vi "SP_OEE_2_test.vi"() -> ()   [LabVIEW 2017] (continued)
                        w9152 = string[] [""]
                        n1667 = Insert Into Array(array=w9162, index (col)=1 ("disabled index (col)"), new element #1=w9152, new element #2=w9152, new element #3=w9152, new element #4=w9152, new element #5=w9152, new element #6=w9152, new element #7=w9152, new element #8=w9152, new element #9=w9153, new element #10=w9154, new element #11=w9155, new element #12=w9156) -> (w9158:string[][])  [unwired: 1 in]
                        n1668 = call "flot graph for month n year.vi"("BD Date"=w9159, "error in (no error)"=w9161, "Count total"=w9155) -> ("error out"=w9160:errorcluster, "Run-Time Status"=w9157:cluster{"Array 2":timestamp[], dbl[]})  [unwired: 7 in]
                        n1669 = local write "Run-Time Status"(w9157) -> ()
                        n1670 = local write "Table"(w9158) -> ()
                      }
                    }
                  }
                  frame "all" {
                  }
                }
              }
            }
          }
          frame "STATION 1" {
            (unwired) "ALL" ("Select Stakeholder")
            n1671 = case shown="\"ALL\"" "ALL" {
              tunnel: w9178 -> [_ w9192 w10652 w12131 w13625 w15132 w16654]
              tunnel: w9177 -> [_ w9191 w10651 w12130 w13624 w15131 w16653]
              tunnel: w9176 -> [_ w9190 w10650 w12129 w13623 w15130 w16652]
              tunnel: w9175 -> [_ w9189 w10649 w12128 w13622 w15129 w16651]
              tunnel: w9174 -> [_ w9188 w10648 w12127 w13621 w15128 w16650]
              tunnel: [_ w9185 _ w12125 _ _ _] -> w9173
              tunnel: [_ w9186 _ w12124 _ _ _] -> w9172
              tunnel: w9170 -> [_ w9184 _ _ _ _ _]
              tunnel: w9169 -> [_ w9183 _ _ _ _ _]
              tunnel: w9168 -> [_ w9182 _ _ _ _ _]
              tunnel: w9167 -> [_ w9181 _ _ _ _ _]
              tunnel: w9166 -> [_ w9180 _ _ _ _ _]
              tunnel: w9165 -> [_ w9179 _ _ _ _ _]
              frame "False", Default {
              }
              frame "ALL" {
                n1672 = local read "Shift"() -> (w9187:string)
                n1673 = case shown="\"ALL\", Default" w9187 {
                  selector: w9187 -> [_ w9568 w9935 w10302 _]
                  tunnel: w9192 -> [w9218 w9577 w9944 w10311 _]
                  tunnel: w9191 -> [w9217 w9576 w9943 w10310 _]
                  tunnel: w9190 -> [w9216 w9575 w9942 w10309 _]
                  tunnel: w9189 -> [w9215 w9574 w9941 w10308 _]
                  tunnel: w9188 -> [w9214 w9573 w9940 w10307 _]
                  tunnel: [w9199 w9553 w9920 w10287 _] -> w9186
                  tunnel: [w9209 w9552 w9919 w10286 _] -> w9185
                  tunnel: w9184 -> [w9207 w9558 w9924 w10293 _]
                  tunnel: w9183 -> [w9206 w9557 w9923 w10292 _]
                  tunnel: w9182 -> [w9205 w9560 w9928 w10295 _]
                  tunnel: w9181 -> [w9204 w9559 w9927 w10294 _]
                  tunnel: w9180 -> [w9202 w9556 w9925 w10290 _]
                  tunnel: w9179 -> [w9201 w9555 w9922 w10289 _]
                  frame "ALL", Default {
                    n1674 = flat-sequence {
                      tunnel: w9218 -> [w9330]
                      tunnel: w9217 -> [w9328]
                      tunnel: [w9314] -> w9308
                      tunnel: [w9329] -> w9307
                      tunnel: w9216 -> [_]
                      tunnel: [w9333] -> w9306
                      tunnel: [w9313] -> w9305
                      tunnel: [w9312] -> w9304
                      tunnel: [w9311] -> w9303
                      tunnel: w9215 -> [w9313]
                      tunnel: w9214 -> [w9312]
                      tunnel: ["Where BREAKDOWN_DATE between '%s'and '%s' and BREAKDOWN_STK_HOLD_ID ='%d' and STATION_ID_CID_TRIGGER =%d "] -> w9302
                      tunnel: [w9311] -> w9301
                      tunnel: w9308 -> [w9394]
                      tunnel: w9307 -> [w9396]
                      tunnel: w9306 -> [w9391]
                      tunnel: w9305 -> [w9390]
                      tunnel: w9304 -> [w9389]
                      tunnel: [w9393] -> w9300
                      tunnel: [w9395] -> w9299
                      tunnel: [w9391] -> w9298
                      tunnel: [w9381] -> w9297
                      tunnel: [w9387] -> w9296
                      tunnel: [w9390] -> w9295
                      tunnel: [w9389] -> w9294
                      tunnel: w9303 -> [w9386]
                      tunnel: [w9386] -> w9293
                      tunnel: w9302 -> [w9383]
                      tunnel: [w9383] -> w9292
                      tunnel: [w9382] -> w9291
                      tunnel: w9301 -> [w9382]
                      tunnel: [w9380] -> w9213
                      tunnel: w9300 -> [w9412]
                      tunnel: w9299 -> [w9410]
                      tunnel: w9298 -> [w9415]
                      tunnel: w9297 -> [w9414]
                      tunnel: w9296 -> [w9413]
                      tunnel: w9295 -> [w9407]
                      tunnel: w9294 -> [w9406]
                      tunnel: [w9415] -> w9290
                      tunnel: [w9414] -> w9289
                      tunnel: [w9413] -> w9288
                      tunnel: [w9411] -> w9287
                      tunnel: [w9404] -> w9286
                      tunnel: [w9403] -> w9285
                      tunnel: [w9408] -> w9284
                      tunnel: [w9407] -> w9283
                      tunnel: [w9406] -> w9282
                      tunnel: w9293 -> [w9402]
                      tunnel: [w9402] -> w9281
                      tunnel: w9292 -> [w9399]
                      tunnel: [w9399] -> w9280
                      tunnel: [w9398] -> w9279
                      tunnel: w9291 -> [w9398]
                      tunnel: w9213 -> [w9397]
                      tunnel: [w9397] -> w9212
                      tunnel: w9290 -> [w9436]
                      tunnel: w9289 -> [w9435]
                      tunnel: w9288 -> [w9434]
                      tunnel: w9287 -> [w9430]
                      tunnel: w9286 -> [w9433]
                      tunnel: w9285 -> [w9432]
                      tunnel: w9284 -> [w9428]
                      tunnel: w9283 -> [w9426]
                      tunnel: w9282 -> [w9425]
                      tunnel: [w9436] -> w9278
                      tunnel: [w9435] -> w9277
                      tunnel: [w9434] -> w9276
                      tunnel: [w9433] -> w9275
                      tunnel: [w9432] -> w9274
                      tunnel: [w9429] -> w9273
                      tunnel: [w9423] -> w9272
                      tunnel: [w9422] -> w9271
                      tunnel: [w9427] -> w9270
                      tunnel: [w9426] -> w9269
                      tunnel: [w9425] -> w9268
                      tunnel: w9281 -> [w9421]
                      tunnel: [w9421] -> w9267
                      tunnel: w9280 -> [w9418]
                      tunnel: [w9418] -> w9266
                      tunnel: [w9417] -> w9265
                      tunnel: w9279 -> [w9417]
                      tunnel: w9212 -> [w9416]
                      tunnel: [w9416] -> w9211
                      tunnel: w9278 -> [w9459]
                      tunnel: w9277 -> [w9458]
                      tunnel: w9276 -> [w9457]
                      tunnel: w9275 -> [w9456]
                      tunnel: w9274 -> [w9455]
                      tunnel: w9273 -> [w9451]
                      tunnel: w9272 -> [w9454]
                      tunnel: w9271 -> [w9453]
                      tunnel: w9270 -> [w9450]
                      tunnel: w9269 -> [w9447]
                      tunnel: w9268 -> [w9446]
                      tunnel: [w9459] -> w9264
                      tunnel: [w9458] -> w9263
                      tunnel: [w9457] -> w9262
                      tunnel: [w9456] -> w9261
                      tunnel: [w9455] -> w9260
                      tunnel: [w9454] -> w9259
                      tunnel: [w9453] -> w9258
                      tunnel: [w9449] -> w9257
                      tunnel: [w9448] -> w9256
                      tunnel: [w9444] -> w9255
                      tunnel: [w9443] -> w9254
                      tunnel: [w9447] -> w9253
                      tunnel: [w9446] -> w9252
                      tunnel: w9267 -> [w9442]
                      tunnel: [w9442] -> w9251
                      tunnel: w9266 -> [w9439]
                      tunnel: [w9439] -> w9250
                      tunnel: [w9438] -> w9249
                      tunnel: w9265 -> [w9438]
                      tunnel: w9211 -> [w9437]
                      tunnel: [w9437] -> w9210
                      tunnel: w9264 -> [w9484]
                      tunnel: w9263 -> [w9483]
                      tunnel: w9262 -> [w9482]
                      tunnel: w9261 -> [w9481]
                      tunnel: w9260 -> [w9480]
                      tunnel: w9259 -> [w9479]
                      tunnel: w9258 -> [w9478]
                      tunnel: w9257 -> [w9472]
                      tunnel: w9256 -> [w9474]
                      tunnel: w9255 -> [w9477]
                      tunnel: w9254 -> [w9476]
                      tunnel: w9253 -> [w9469]
                      tunnel: w9252 -> [w9470]
                      tunnel: [w9484] -> w9248
                      tunnel: [w9483] -> w9247
                      tunnel: [w9482] -> w9246
                      tunnel: [w9481] -> w9245
                      tunnel: [w9480] -> w9244
                      tunnel: [w9479] -> w9243
                      tunnel: [w9478] -> w9242
                      tunnel: [w9477] -> w9241
                      tunnel: [w9476] -> w9240
                      tunnel: [w9473] -> w9239
                      tunnel: [w9471] -> w9238
                      tunnel: [w9467] -> w9237
                      tunnel: [w9465] -> w9236
                      tunnel: w9251 -> [w9466]
                      tunnel: w9250 -> [w9462]
                      tunnel: [w9461] -> w9235
                      tunnel: w9249 -> [w9461]
                      tunnel: w9210 -> [w9460]
                      tunnel: w9248 -> [w9511]
                      tunnel: w9247 -> [w9504]
                      tunnel: w9246 -> [w9495]
                      tunnel: w9245 -> [w9503]
                      tunnel: w9244 -> [w9493]
                      tunnel: w9243 -> [w9502]
                      tunnel: w9242 -> [w9491]
                      tunnel: w9241 -> [w9501]
                      tunnel: w9240 -> [w9489]
                      tunnel: w9239 -> [w9525]
                      tunnel: w9238 -> [w9524]
                      tunnel: w9237 -> [w9500]
                      tunnel: w9236 -> [w9487]
                      tunnel: [w9525] -> w9234
                      tunnel: [w9524] -> w9233
                      tunnel: [w9518] -> w9232
                      tunnel: [w9511] -> w9231
                      tunnel: [w9510] -> w9230
                      tunnel: [w9509] -> w9229
                      tunnel: [w9508] -> w9228
                      tunnel: [w9507] -> w9227
                      tunnel: [w9506] -> w9226
                      tunnel: [w9505] -> w9225
                      tunnel: [w9504] -> w9224
                      tunnel: [w9503] -> w9223
                      tunnel: [w9502] -> w9222
                      tunnel: [w9501] -> w9221
                      tunnel: [w9500] -> w9220
                      tunnel: [w9485] -> w9219
                      tunnel: w9235 -> [w9485]
                      tunnel: [w9545] -> w9200
                      tunnel: [w9531] -> w9209
                      tunnel: w9234 -> [w9532]
                      tunnel: w9233 -> [w9545]
                      tunnel: w9232 -> [w9530]
                      tunnel: w9231 -> [w9543]
                      tunnel: w9230 -> [w9541]
                      tunnel: w9229 -> [w9539]
                      tunnel: w9228 -> [w9537]
                      tunnel: w9227 -> [w9535]
                      tunnel: w9226 -> [w9533]
                      tunnel: w9225 -> [w9526]
                      tunnel: w9224 -> [w9542]
                      tunnel: w9223 -> [w9540]
                      tunnel: w9222 -> [w9538]
                      tunnel: w9221 -> [w9536]
                      tunnel: w9220 -> [w9534]
                      tunnel: w9219 -> [w9529]
                      tunnel: [w9526] -> w9203
                      frame #0 {
                        w9321 = "%Y-%m-%d" ("time format string (%c)")
                        n1675 = property on="Table" class="Tbl (strict)"("Visible"=TRUE) -> ()  [unwired: 2 in, 2 out]
                        n1676 = Format Date/Time String(time format string (%c)=w9321, seconds (now)=w9313) -> (date/time string=w9322:string)  [unwired: 1 in]
                        n1677 = Format Date/Time String(time format string (%c)=w9321, seconds (now)=w9312) -> (date/time string=w9320:string)  [unwired: 1 in]
                        n1678 = Format Into String(format string="Where BREAKDOWN_DATE between '%s' and '%s' ", w9322, w9320) -> (resulting string=w9319:string)  [unwired: 2 in, 1 out]
                        n1679 = call <vilib>:"DB Tools Select Data.vi"("condition"=w9319, "error in (no error)"=w9328, "columns"=string[] ["BREAKDOWN_DATE"], "table"="STATION_1_LOG_HISTORY", "connection reference"=w9330) -> ("error out"=w9315:errorcluster, "data"=w9318:variant[][], "connection reference out"=w9329:T2)  [unwired: 1 in]
                        n1680 = property on="Table 2" class="Tbl (strict)"("Visible"=FALSE) -> ()  [unwired: 2 in, 2 out]
                        n1681 = xnode "Database Variant To Data"("database variant"=w9318, "error in (no error)"=w9315, "type"=string[][] [] ("Elements Found")) -> ("data"=w9316:string[][], "error out"=w9314:errorcluster)
                        n1682 = Index Array(array=w9316, index (col)=0 ("disabled index (col)")) -> (element=w9324:string[])  [unwired: 1 in]
                        n1683 = call "Search_1d_array_element.vi"("Count in"=string[] [] ("Elements Found"), "BD Date"=w9324, "Elements Found in"=string[] [] ("Elements Found")) -> ("Elements Found out"=w9311:string[])  [unwired: 4 in, 2 out]
                        n1684 = Build Array(w9311) -> (w9334:string[][])
                        n1685 = Transpose 2D Array(2D array=w9334) -> (transposed array=w9333:string[][])
                      }
                      frame #1 {
                        w9380 = 1 ("STATION_ID_CID_TRIGGER")
                        n1686 = call "Stack_holderwise_total_bd_count_&_duration_ST1.vi"("Refnum in"=w9396, "BREAKDOWN_STK_HOLD_ID"=1, "condition"=w9383, "Form Date"=w9390, "To Date"=w9389, "error in (no error)"=w9394, "STATION_ID_CID_TRIGGER"=w9380) -> ("Refnum out"=w9395:T2, "Count out"=w9388:string[], "appended array"=w9385:dbl[], "error out"=w9393:errorcluster)  [unwired: 5 in]
                        n1687 = call "NUMERIC TO STRING.vi"("appended array"=w9385) -> ("Array"=w9384:string[])  [unwired: 4 in]
                        n1688 = call "Insert_empty_element_with_zero.vi"("searched date"=w9388, "fixed date"=w9386) -> ("O/P"=w9381:string[])  [unwired: 9 in]
                        n1689 = call "Insert_empty_element_with_zero.vi"("searched date"=w9384, "fixed date"=w9386) -> ("O/P"=w9387:string[])  [unwired: 9 in]
                      }
                      frame #2 {
                        n1690 = call "Stack_holderwise_total_bd_count_&_duration_ST1.vi"("Refnum in"=w9410, "BREAKDOWN_STK_HOLD_ID"=2, "condition"=w9399, "Form Date"=w9407, "To Date"=w9406, "error in (no error)"=w9412, "STATION_ID_CID_TRIGGER"=w9397) -> ("Refnum out"=w9408:T2, "Count out"=w9405:string[], "appended array"=w9401:dbl[], "error out"=w9411:errorcluster)  [unwired: 5 in]
                        n1691 = call "Insert_empty_element_with_zero.vi"("searched date"=w9405, "fixed date"=w9402) -> ("O/P"=w9404:string[])  [unwired: 9 in]
                        n1692 = call "NUMERIC TO STRING.vi"("appended array"=w9401) -> ("Array"=w9400:string[])  [unwired: 4 in]
                        n1693 = call "Insert_empty_element_with_zero.vi"("searched date"=w9400, "fixed date"=w9402) -> ("O/P"=w9403:string[])  [unwired: 9 in]
                      }
                      frame #3 {
                        n1694 = call "Stack_holderwise_total_bd_count_&_duration_ST1.vi"("Refnum in"=w9428, "BREAKDOWN_STK_HOLD_ID"=3, "condition"=w9418, "Form Date"=w9426, "To Date"=w9425, "error in (no error)"=w9430, "STATION_ID_CID_TRIGGER"=w9416) -> ("Refnum out"=w9427:T2, "Count out"=w9424:string[], "appended array"=w9420:dbl[], "error out"=w9429:errorcluster)  [unwired: 5 in]
                        n1695 = call "Insert_empty_element_with_zero.vi"("searched date"=w9424, "fixed date"=w9421) -> ("O/P"=w9423:string[])  [unwired: 9 in]
                        n1696 = call "NUMERIC TO STRING.vi"("appended array"=w9420) -> ("Array"=w9419:string[])  [unwired: 4 in]
                        n1697 = call "Insert_empty_element_with_zero.vi"("searched date"=w9419, "fixed date"=w9421) -> ("O/P"=w9422:string[])  [unwired: 9 in]
                      }
                      frame #4 {
                        n1698 = call "Stack_holderwise_total_bd_count_&_duration_ST1.vi"("Refnum in"=w9450, "BREAKDOWN_STK_HOLD_ID"=4, "condition"=w9439, "Form Date"=w9447, "To Date"=w9446, "error in (no error)"=w9451, "STATION_ID_CID_TRIGGER"=w9437) -> ("Refnum out"=w9449:T2, "Count out"=w9445:string[], "appended array"=w9441:dbl[], "error out"=w9448:errorcluster)  [unwired: 5 in]
                        n1699 = call "Insert_empty_element_with_zero.vi"("searched date"=w9445, "fixed date"=w9442) -> ("O/P"=w9444:string[])  [unwired: 9 in]
                        n1700 = call "NUMERIC TO STRING.vi"("appended array"=w9441) -> ("Array"=w9440:string[])  [unwired: 4 in]
                        n1701 = call "Insert_empty_element_with_zero.vi"("searched date"=w9440, "fixed date"=w9442) -> ("O/P"=w9443:string[])  [unwired: 9 in]
                      }
                      frame #5 {
                        n1702 = call "Stack_holderwise_total_bd_count_&_duration_ST1.vi"("Refnum in"=w9472, "BREAKDOWN_STK_HOLD_ID"=5, "condition"=w9462, "Form Date"=w9469, "To Date"=w9470, "error in (no error)"=w9474, "STATION_ID_CID_TRIGGER"=w9460) -> ("Refnum out"=w9471:T2, "Count out"=w9468:string[], "appended array"=w9464:dbl[], "error out"=w9473:errorcluster)  [unwired: 5 in]
                        n1703 = call "NUMERIC TO STRING.vi"("appended array"=w9464) -> ("Array"=w9463:string[])  [unwired: 4 in]
                        n1704 = call "Insert_empty_element_with_zero.vi"("searched date"=w9468, "fixed date"=w9466) -> ("O/P"=w9467:string[])  [unwired: 9 in]
                        n1705 = call "Insert_empty_element_with_zero.vi"("searched date"=w9463, "fixed date"=w9466) -> ("O/P"=w9465:string[])  [unwired: 9 in]
                      }
                      frame #6 {
                        n1706 = call "String to numeric.vi"("Array"=w9495) -> ("Array 2"=w9494:dbl[])  [unwired: 4 in]
                        n1707 = call "String to numeric.vi"("Array"=w9493) -> ("Array 2"=w9492:dbl[])  [unwired: 4 in]
                        n1708 = call "String to numeric.vi"("Array"=w9491) -> ("Array 2"=w9490:dbl[])  [unwired: 4 in]
                        n1709 = call "String to numeric.vi"("Array"=w9489) -> ("Array 2"=w9488:dbl[])  [unwired: 4 in]
                        n1710 = call "String to numeric.vi"("Array"=w9487) -> ("Array 2"=w9486:dbl[])  [unwired: 4 in]
                        n1711 = Decimal String To Number(string=w9500) -> (number=w9519:i32[])  [unwired: 2 in, 1 out]
                        n1712 = Decimal String To Number(string=w9501) -> (number=w9520:i32[])  [unwired: 2 in, 1 out]
                        n1713 = Decimal String To Number(string=w9502) -> (number=w9521:i32[])  [unwired: 2 in, 1 out]
                        n1714 = Decimal String To Number(string=w9503) -> (number=w9522:i32[])  [unwired: 2 in, 1 out]
                        n1715 = Decimal String To Number(string=w9504) -> (number=w9517:i32[])  [unwired: 2 in, 1 out]
                        n1716 = Compound Arithmetic op=ADD(w9494, w9492, w9490, w9488, w9486) -> (w9497:dbl[])
                        n1717 = Build Array(w9495) -> (w9516:string[][])
                        n1718 = Build Array(w9493) -> (w9515:string[][])
                        n1719 = Build Array(w9491) -> (w9514:string[][])
                        n1720 = Build Array(w9489) -> (w9513:string[][])
                        n1721 = Build Array(w9487) -> (w9512:string[][])
                        n1722 = Number To Fractional String(number=w9497, precision (6)=i16 2) -> (F-format string=w9496:string[])  [unwired: 2 in]
                        n1723 = Compound Arithmetic op=ADD(w9519, w9520, w9521, w9522, w9517) -> (w9523:i32[])
                        n1724 = Transpose 2D Array(2D array=w9516) -> (transposed array=w9510:string[][])
                        n1725 = Transpose 2D Array(2D array=w9515) -> (transposed array=w9509:string[][])
                        n1726 = Transpose 2D Array(2D array=w9514) -> (transposed array=w9508:string[][])
                        n1727 = Transpose 2D Array(2D array=w9513) -> (transposed array=w9507:string[][])
                        n1728 = Transpose 2D Array(2D array=w9512) -> (transposed array=w9506:string[][])
                        n1729 = Number To Decimal String(number=w9523) -> (decimal integer string=w9518:string[])  [unwired: 1 in]
                        n1730 = Build Array(w9496) -> (w9499:string[][])
                        n1731 = Transpose 2D Array(2D array=w9499) -> (transposed array=w9505:string[][])
                      }
                      frame #7 {
                        n1732 = Insert Into Array(array=w9543, index (col)=1 ("disabled index (col)"), new element #1=w9542, new element #2=w9541, new element #3=w9540, new element #4=w9539, new element #5=w9538, new element #6=w9537, new element #7=w9536, new element #8=w9535, new element #9=w9534, new element #10=w9533, new element #11=w9530, new element #12=w9526) -> (w9528:string[][])  [unwired: 1 in]
                        n1733 = call "flot graph for month n year.vi"("BD Date"=w9529, "error in (no error)"=w9532, "Count total"=w9530) -> ("error out"=w9531:errorcluster, "Run-Time Status"=w9527:cluster{"Array 2":timestamp[], dbl[]})  [unwired: 7 in]
                        n1734 = local write "Run-Time Status"(w9527) -> ()
                        n1735 = local write "Table"(w9528) -> ()
                      }
                    }
                    n1736 = call "OEE_PART_1.vi"("CYCLE TIME"=w9204, "ACTUAL PROD TIME"=w9205, "BREAKDOWN TOTAL TIME"=w9203) -> ("Numeric"=w9194:i32, "CAPACITY"=w9193:dbl, "ACTUAL TIME"=w9195:i32)  [unwired: 5 in, 1 out]
                    n1737 = call "OEE_PART_2_P.vi"("Refnum in"=w9200, "Shift"=w9202, "String"="ALL", "Select Station"=w9201, "Form Date"=w9207, "To Date"=w9206, "AVAILABLILITY TIME"=w9195, "CAPACITY"=w9193) -> ("Refnum out"=w9199:T2, "QUALITY"=w9198:dbl, "OEE"=w9196:dbl, "PERFORMANCE"=w9197:dbl)  [unwired: 2 in, 2 out]
                    n1738 = local write "PERFORMANCE"(w9197) -> ()
                    n1739 = local write "QUALITY"(w9198) -> ()
                    n1740 = local write "OEE"(w9196) -> ()
                    n1741 = local write "AVAILABLILITY TIME(MIN)"(w9195) -> ()
                    n1742 = local write "IDEAL CYCLE TIME"(w9194) -> ()
                    n1743 = local write "CAPACITY"(w9193) -> ()
                  }
                  frame "1" {
                    n1744 = flat-sequence {
                      tunnel: w9577 -> [w9692]
                      tunnel: w9576 -> [w9690]
                      tunnel: [w9676] -> w9667
                      tunnel: [w9691] -> w9666
                      tunnel: w9575 -> [_]
                      tunnel: [w9695] -> w9665
                      tunnel: [w9675] -> w9664
                      tunnel: [w9674] -> w9663
                      tunnel: [w9672] -> w9662
                      tunnel: w9574 -> [w9675]
                      tunnel: w9573 -> [w9674]
                      tunnel: ["Where BREAKDOWN_DATE between '%s'and '%s' and BREAKDOWN_STK_HOLD_ID ='%d' and  SHIFT_ID = '%d' and STATION_ID_CID_TRIGGER =%d  "] -> w9661
                      tunnel: [w9672] -> w9660
                      tunnel: w9568 -> [w9670]
                      tunnel: [1 ("BREAKDOWN_STK_HOLD_ID")] -> w9567
                      tunnel: w9667 -> [w9757]
                      tunnel: w9666 -> [w9759]
                      tunnel: w9665 -> [w9754]
                      tunnel: w9664 -> [w9753]
                      tunnel: w9663 -> [w9752]
                      tunnel: [w9756] -> w9659
                      tunnel: [w9758] -> w9658
                      tunnel: [w9754] -> w9657
                      tunnel: [w9744] -> w9656
                      tunnel: [w9750] -> w9655
                      tunnel: [w9753] -> w9654
                      tunnel: [w9752] -> w9653
                      tunnel: w9662 -> [w9749]
                      tunnel: [w9749] -> w9652
                      tunnel: w9661 -> [w9746]
                      tunnel: [w9746] -> w9651
                      tunnel: [w9745] -> w9650
                      tunnel: w9660 -> [w9745]
                      tunnel: w9568 -> [w9743]
                      tunnel: [w9743] -> w9572
                      tunnel: w9567 -> [w9742]
                      tunnel: [w9742] -> w9566
                      tunnel: w9659 -> [w9776]
                      tunnel: w9658 -> [w9774]
                      tunnel: w9657 -> [w9779]
                      tunnel: w9656 -> [w9778]
                      tunnel: w9655 -> [w9777]
                      tunnel: w9654 -> [w9771]
                      tunnel: w9653 -> [w9770]
                      tunnel: [w9779] -> w9649
                      tunnel: [w9778] -> w9648
                      tunnel: [w9777] -> w9647
                      tunnel: [w9775] -> w9646
                      tunnel: [w9768] -> w9645
                      tunnel: [w9767] -> w9644
                      tunnel: [w9772] -> w9643
                      tunnel: [w9771] -> w9642
                      tunnel: [w9770] -> w9641
                      tunnel: w9652 -> [w9766]
                      tunnel: [w9766] -> w9640
                      tunnel: w9651 -> [w9763]
                      tunnel: [w9763] -> w9639
                      tunnel: [w9762] -> w9638
                      tunnel: w9650 -> [w9762]
                      tunnel: w9572 -> [w9761]
                      tunnel: [w9761] -> w9571
                      tunnel: w9566 -> [w9760]
                      tunnel: [w9760] -> w9565
                      tunnel: w9649 -> [w9801]
                      tunnel: w9648 -> [w9800]
                      tunnel: w9647 -> [w9799]
                      tunnel: w9646 -> [w9795]
                      tunnel: w9645 -> [w9798]
                      tunnel: w9644 -> [w9797]
                      tunnel: w9643 -> [w9793]
                      tunnel: w9642 -> [w9791]
                      tunnel: w9641 -> [w9790]
                      tunnel: [w9801] -> w9637
                      tunnel: [w9800] -> w9636
                      tunnel: [w9799] -> w9635
                      tunnel: [w9798] -> w9634
                      tunnel: [w9797] -> w9633
                      tunnel: [w9794] -> w9632
                      tunnel: [w9788] -> w9631
                      tunnel: [w9787] -> w9630
                      tunnel: [w9792] -> w9629
                      tunnel: [w9791] -> w9628
                      tunnel: [w9790] -> w9627
                      tunnel: w9640 -> [w9786]
                      tunnel: [w9786] -> w9626
                      tunnel: w9639 -> [w9783]
                      tunnel: [w9783] -> w9625
                      tunnel: [w9782] -> w9624
                      tunnel: w9638 -> [w9782]
                      tunnel: w9571 -> [w9781]
                      tunnel: [w9781] -> w9570
                      tunnel: w9565 -> [w9780]
                      tunnel: [w9780] -> w9564
                      tunnel: w9637 -> [w9825]
                      tunnel: w9636 -> [w9824]
                      tunnel: w9635 -> [w9823]
                      tunnel: w9634 -> [w9822]
                      tunnel: w9633 -> [w9821]
                      tunnel: w9632 -> [w9817]
                      tunnel: w9631 -> [w9820]
                      tunnel: w9630 -> [w9819]
                      tunnel: w9629 -> [w9816]
                      tunnel: w9628 -> [w9813]
                      tunnel: w9627 -> [w9812]
                      tunnel: [w9825] -> w9623
                      tunnel: [w9824] -> w9622
                      tunnel: [w9823] -> w9621
                      tunnel: [w9822] -> w9620
                      tunnel: [w9821] -> w9619
                      tunnel: [w9820] -> w9618
                      tunnel: [w9819] -> w9617
                      tunnel: [w9815] -> w9616
                      tunnel: [w9814] -> w9615
                      tunnel: [w9810] -> w9614
                      tunnel: [w9809] -> w9613
                      tunnel: [w9813] -> w9612
                      tunnel: [w9812] -> w9611
                      tunnel: w9626 -> [w9808]
                      tunnel: [w9808] -> w9610
                      tunnel: w9625 -> [w9805]
                      tunnel: [w9805] -> w9609
                      tunnel: [w9804] -> w9608
                      tunnel: w9624 -> [w9804]
                      tunnel: w9570 -> [w9803]
                      tunnel: [w9803] -> w9569
                      tunnel: w9564 -> [w9802]
                      tunnel: [w9802] -> w9563
                      tunnel: w9623 -> [w9851]
                      tunnel: w9622 -> [w9850]
                      tunnel: w9621 -> [w9849]
                      tunnel: w9620 -> [w9848]
                      tunnel: w9619 -> [w9847]
                      tunnel: w9618 -> [w9846]
                      tunnel: w9617 -> [w9845]
                      tunnel: w9616 -> [w9839]
                      tunnel: w9615 -> [w9841]
                      tunnel: w9614 -> [w9844]
                      tunnel: w9613 -> [w9843]
                      tunnel: w9612 -> [w9836]
                      tunnel: w9611 -> [w9837]
                      tunnel: [w9851] -> w9607
                      tunnel: [w9850] -> w9606
                      tunnel: [w9849] -> w9605
                      tunnel: [w9848] -> w9604
                      tunnel: [w9847] -> w9603
                      tunnel: [w9846] -> w9602
                      tunnel: [w9845] -> w9601
                      tunnel: [w9844] -> w9600
                      tunnel: [w9843] -> w9599
                      tunnel: [w9840] -> w9598
                      tunnel: [w9838] -> w9597
                      tunnel: [w9834] -> w9596
                      tunnel: [w9832] -> w9595
                      tunnel: w9610 -> [w9833]
                      tunnel: w9609 -> [w9829]
                      tunnel: [w9828] -> w9594
                      tunnel: w9608 -> [w9828]
                      tunnel: w9569 -> [w9827]
                      tunnel: w9563 -> [w9826]
                      tunnel: w9607 -> [w9878]
                      tunnel: w9606 -> [w9871]
                      tunnel: w9605 -> [w9862]
                      tunnel: w9604 -> [w9870]
                      tunnel: w9603 -> [w9860]
                      tunnel: w9602 -> [w9869]
                      tunnel: w9601 -> [w9858]
                      tunnel: w9600 -> [w9868]
                      tunnel: w9599 -> [w9856]
                      tunnel: w9598 -> [w9892]
                      tunnel: w9597 -> [w9891]
                      tunnel: w9596 -> [w9867]
                      tunnel: w9595 -> [w9854]
                      tunnel: [w9892] -> w9593
                      tunnel: [w9891] -> w9592
                      tunnel: [w9885] -> w9591
                      tunnel: [w9878] -> w9590
                      tunnel: [w9877] -> w9589
                      tunnel: [w9876] -> w9588
                      tunnel: [w9875] -> w9587
                      tunnel: [w9874] -> w9586
                      tunnel: [w9873] -> w9585
                      tunnel: [w9872] -> w9584
                      tunnel: [w9871] -> w9583
                      tunnel: [w9870] -> w9582
                      tunnel: [w9869] -> w9581
                      tunnel: [w9868] -> w9580
                      tunnel: [w9867] -> w9579
                      tunnel: [w9852] -> w9578
                      tunnel: w9594 -> [w9852]
                      tunnel: [w9912] -> w9554
                      tunnel: [w9898] -> w9552
                      tunnel: w9593 -> [w9899]
                      tunnel: w9592 -> [w9912]
                      tunnel: w9591 -> [w9897]
                      tunnel: w9590 -> [w9910]
                      tunnel: w9589 -> [w9908]
                      tunnel: w9588 -> [w9906]
                      tunnel: w9587 -> [w9904]
                      tunnel: w9586 -> [w9902]
                      tunnel: w9585 -> [w9900]
                      tunnel: w9584 -> [w9893]
                      tunnel: w9583 -> [w9909]
                      tunnel: w9582 -> [w9907]
                      tunnel: w9581 -> [w9905]
                      tunnel: w9580 -> [w9903]
                      tunnel: w9579 -> [w9901]
                      tunnel: w9578 -> [w9896]
                      tunnel: [w9893] -> w9561
                      frame #0 {
                        w9683 = "%Y-%m-%d" ("time format string (%c)")
                        n1745 = Decimal String To Number(string=w9670) -> (number=w9669:i32)  [unwired: 2 in, 1 out]
                        n1746 = property on="Table" class="Tbl (strict)"("Visible"=TRUE) -> ()  [unwired: 2 in, 2 out]
                        n1747 = Format Date/Time String(time format string (%c)=w9683, seconds (now)=w9675) -> (date/time string=w9684:string)  [unwired: 1 in]
                        n1748 = Format Date/Time String(time format string (%c)=w9683, seconds (now)=w9674) -> (date/time string=w9682:string)  [unwired: 1 in]
                        n1749 = Format Into String(format string="Where BREAKDOWN_DATE between '%s' and '%s' and  SHIFT_ID = '%d'  ", w9684, w9682, w9669) -> (resulting string=w9681:string)  [unwired: 2 in, 1 out]
                        n1750 = call <vilib>:"DB Tools Select Data.vi"("condition"=w9681, "error in (no error)"=w9690, "columns"=string[] ["BREAKDOWN_DATE"], "table"="STATION_1_LOG_HISTORY", "connection reference"=w9692) -> ("error out"=w9677:errorcluster, "data"=w9680:variant[][], "connection reference out"=w9691:T2)  [unwired: 1 in]
                        n1751 = property on="Table 2" class="Tbl (strict)"("Visible"=FALSE) -> ()  [unwired: 2 in, 2 out]
                        n1752 = xnode "Database Variant To Data"("database variant"=w9680, "error in (no error)"=w9677, "type"=string[][] [] ("Elements Found")) -> ("data"=w9678:string[][], "error out"=w9676:errorcluster)
                        n1753 = Index Array(array=w9678, index (col)=0 ("disabled index (col)")) -> (element=w9686:string[])  [unwired: 1 in]
                        n1754 = call "Search_1d_array_element.vi"("Count in"=string[] [] ("Elements Found"), "BD Date"=w9686, "Elements Found in"=string[] [] ("Elements Found")) -> ("Elements Found out"=w9672:string[])  [unwired: 4 in, 2 out]
                        n1755 = Build Array(w9672) -> (w9696:string[][])
                        n1756 = Transpose 2D Array(2D array=w9696) -> (transposed array=w9695:string[][])
                      }
                      frame #1 {
                        n1757 = call "Stack_holderwise_total_bd_count_&_duration_3_for_stationwise.vi"("Refnum in"=w9759, "BREAKDOWN_STK_HOLD_ID"=1, "condition"=w9746, "Form Date"=w9753, "To Date"=w9752, "error in (no error)"=w9757, "STATION_ID_CID_TRIGGER"=w9742, "Shift"=w9743) -> ("Refnum out"=w9758:T2, "Count out"=w9751:string[], "appended array"=w9748:dbl[], "error out"=w9756:errorcluster)  [unwired: 4 in]
                        n1758 = call "NUMERIC TO STRING.vi"("appended array"=w9748) -> ("Array"=w9747:string[])  [unwired: 4 in]
                        n1759 = call "Insert_empty_element_with_zero.vi"("searched date"=w9751, "fixed date"=w9749) -> ("O/P"=w9744:string[])  [unwired: 9 in]
                        n1760 = call "Insert_empty_element_with_zero.vi"("searched date"=w9747, "fixed date"=w9749) -> ("O/P"=w9750:string[])  [unwired: 9 in]
                      }
                      frame #2 {
                        n1761 = call "Stack_holderwise_total_bd_count_&_duration_3_for_stationwise.vi"("Refnum in"=w9774, "BREAKDOWN_STK_HOLD_ID"=2, "condition"=w9763, "Form Date"=w9771, "To Date"=w9770, "error in (no error)"=w9776, "STATION_ID_CID_TRIGGER"=w9760, "Shift"=w9761) -> ("Refnum out"=w9772:T2, "Count out"=w9769:string[], "appended array"=w9765:dbl[], "error out"=w9775:errorcluster)  [unwired: 4 in]
                        n1762 = call "Insert_empty_element_with_zero.vi"("searched date"=w9769, "fixed date"=w9766) -> ("O/P"=w9768:string[])  [unwired: 9 in]
                        n1763 = call "NUMERIC TO STRING.vi"("appended array"=w9765) -> ("Array"=w9764:string[])  [unwired: 4 in]
                        n1764 = call "Insert_empty_element_with_zero.vi"("searched date"=w9764, "fixed date"=w9766) -> ("O/P"=w9767:string[])  [unwired: 9 in]
                      }
                      frame #3 {
                        n1765 = call "Stack_holderwise_total_bd_count_&_duration_3_for_stationwise.vi"("Refnum in"=w9793, "BREAKDOWN_STK_HOLD_ID"=3, "condition"=w9783, "Form Date"=w9791, "To Date"=w9790, "error in (no error)"=w9795, "STATION_ID_CID_TRIGGER"=w9780, "Shift"=w9781) -> ("Refnum out"=w9792:T2, "Count out"=w9789:string[], "appended array"=w9785:dbl[], "error out"=w9794:errorcluster)  [unwired: 4 in]
                        n1766 = call "Insert_empty_element_with_zero.vi"("searched date"=w9789, "fixed date"=w9786) -> ("O/P"=w9788:string[])  [unwired: 9 in]
                        n1767 = call "NUMERIC TO STRING.vi"("appended array"=w9785) -> ("Array"=w9784:string[])  [unwired: 4 in]
                        n1768 = call "Insert_empty_element_with_zero.vi"("searched date"=w9784, "fixed date"=w9786) -> ("O/P"=w9787:string[])  [unwired: 9 in]
                      }
                      frame #4 {
                        n1769 = call "Stack_holderwise_total_bd_count_&_duration_3_for_stationwise.vi"("Refnum in"=w9816, "BREAKDOWN_STK_HOLD_ID"=4, "condition"=w9805, "Form Date"=w9813, "To Date"=w9812, "error in (no error)"=w9817, "STATION_ID_CID_TRIGGER"=w9802, "Shift"=w9803) -> ("Refnum out"=w9815:T2, "Count out"=w9811:string[], "appended array"=w9807:dbl[], "error out"=w9814:errorcluster)  [unwired: 4 in]
                        n1770 = call "Insert_empty_element_with_zero.vi"("searched date"=w9811, "fixed date"=w9808) -> ("O/P"=w9810:string[])  [unwired: 9 in]
                        n1771 = call "NUMERIC TO STRING.vi"("appended array"=w9807) -> ("Array"=w9806:string[])  [unwired: 4 in]
                        n1772 = call "Insert_empty_element_with_zero.vi"("searched date"=w9806, "fixed date"=w9808) -> ("O/P"=w9809:string[])  [unwired: 9 in]
                      }
                      frame #5 {
                        n1773 = call "Stack_holderwise_total_bd_count_&_duration_3_for_stationwise.vi"("Refnum in"=w9839, "BREAKDOWN_STK_HOLD_ID"=5, "condition"=w9829, "Form Date"=w9836, "To Date"=w9837, "error in (no error)"=w9841, "STATION_ID_CID_TRIGGER"=w9826, "Shift"=w9827) -> ("Refnum out"=w9838:T2, "Count out"=w9835:string[], "appended array"=w9831:dbl[], "error out"=w9840:errorcluster)  [unwired: 4 in]
                        n1774 = call "NUMERIC TO STRING.vi"("appended array"=w9831) -> ("Array"=w9830:string[])  [unwired: 4 in]
                        n1775 = call "Insert_empty_element_with_zero.vi"("searched date"=w9835, "fixed date"=w9833) -> ("O/P"=w9834:string[])  [unwired: 9 in]
                        n1776 = call "Insert_empty_element_with_zero.vi"("searched date"=w9830, "fixed date"=w9833) -> ("O/P"=w9832:string[])  [unwired: 9 in]
                      }
                      frame #6 {
                        n1777 = call "String to numeric.vi"("Array"=w9862) -> ("Array 2"=w9861:dbl[])  [unwired: 4 in]
                        n1778 = call "String to numeric.vi"("Array"=w9860) -> ("Array 2"=w9859:dbl[])  [unwired: 4 in]
                        n1779 = call "String to numeric.vi"("Array"=w9858) -> ("Array 2"=w9857:dbl[])  [unwired: 4 in]
                        n1780 = call "String to numeric.vi"("Array"=w9856) -> ("Array 2"=w9855:dbl[])  [unwired: 4 in]
                        n1781 = call "String to numeric.vi"("Array"=w9854) -> ("Array 2"=w9853:dbl[])  [unwired: 4 in]
                        n1782 = Decimal String To Number(string=w9867) -> (number=w9886:i32[])  [unwired: 2 in, 1 out]
                        n1783 = Decimal String To Number(string=w9868) -> (number=w9887:i32[])  [unwired: 2 in, 1 out]
                        n1784 = Decimal String To Number(string=w9869) -> (number=w9888:i32[])  [unwired: 2 in, 1 out]
                        n1785 = Decimal String To Number(string=w9870) -> (number=w9889:i32[])  [unwired: 2 in, 1 out]
                        n1786 = Decimal String To Number(string=w9871) -> (number=w9884:i32[])  [unwired: 2 in, 1 out]
                        n1787 = Compound Arithmetic op=ADD(w9861, w9859, w9857, w9855, w9853) -> (w9864:dbl[])
                        n1788 = Build Array(w9862) -> (w9883:string[][])
                        n1789 = Build Array(w9860) -> (w9882:string[][])
                        n1790 = Build Array(w9858) -> (w9881:string[][])
                        n1791 = Build Array(w9856) -> (w9880:string[][])
                        n1792 = Build Array(w9854) -> (w9879:string[][])
                        n1793 = Number To Fractional String(number=w9864, precision (6)=i16 2) -> (F-format string=w9863:string[])  [unwired: 2 in]
                        n1794 = Compound Arithmetic op=ADD(w9886, w9887, w9888, w9889, w9884) -> (w9890:i32[])
                        n1795 = Transpose 2D Array(2D array=w9883) -> (transposed array=w9877:string[][])
                        n1796 = Transpose 2D Array(2D array=w9882) -> (transposed array=w9876:string[][])
                        n1797 = Transpose 2D Array(2D array=w9881) -> (transposed array=w9875:string[][])
                        n1798 = Transpose 2D Array(2D array=w9880) -> (transposed array=w9874:string[][])
                        n1799 = Transpose 2D Array(2D array=w9879) -> (transposed array=w9873:string[][])
                        n1800 = Number To Decimal String(number=w9890) -> (decimal integer string=w9885:string[])  [unwired: 1 in]
                        n1801 = Build Array(w9863) -> (w9866:string[][])
                        n1802 = Transpose 2D Array(2D array=w9866) -> (transposed array=w9872:string[][])
                      }
                      frame #7 {
                        n1803 = Insert Into Array(array=w9910, index (col)=1 ("disabled index (col)"), new element #1=w9909, new element #2=w9908, new element #3=w9907, new element #4=w9906, new element #5=w9905, new element #6=w9904, new element #7=w9903, new element #8=w9902, new element #9=w9901, new element #10=w9900, new element #11=w9897, new element #12=w9893) -> (w9895:string[][])  [unwired: 1 in]
                        n1804 = call "flot graph for month n year.vi"("BD Date"=w9896, "error in (no error)"=w9899, "Count total"=w9897) -> ("error out"=w9898:errorcluster, "Run-Time Status"=w9894:cluster{"Array 2":timestamp[], dbl[]})  [unwired: 7 in]
                        n1805 = local write "Run-Time Status"(w9894) -> ()
                        n1806 = local write "Table"(w9895) -> ()
                      }
                    }
                    n1807 = call "OEE_PART_1.vi"("CYCLE TIME"=w9559, "ACTUAL PROD TIME"=w9560, "BREAKDOWN TOTAL TIME"=w9561) -> ("Numeric"=w9547:i32, "CAPACITY"=w9546:dbl, "ACTUAL TIME"=w9548:i32)  [unwired: 5 in, 1 out]
                    n1808 = call "OEE_PART_2_P.vi"("Refnum in"=w9554, "Shift"=w9556, "String"="ALL", "Select Station"=w9555, "Form Date"=w9558, "To Date"=w9557, "AVAILABLILITY TIME"=w9548, "CAPACITY"=w9546) -> ("Refnum out"=w9553:T2, "QUALITY"=w9551:dbl, "OEE"=w9549:dbl, "PERFORMANCE"=w9550:dbl)  [unwired: 2 in, 2 out]
                    n1809 = local write "PERFORMANCE"(w9550) -> ()
                    n1810 = local write "QUALITY"(w9551) -> ()
                    n1811 = local write "OEE"(w9549) -> ()
                    n1812 = local write "AVAILABLILITY TIME(MIN)"(w9548) -> ()
                    n1813 = local write "IDEAL CYCLE TIME"(w9547) -> ()
                    n1814 = local write "CAPACITY"(w9546) -> ()
                  }
                  frame "2" {
                    n1815 = flat-sequence {
                      tunnel: w9944 -> [w10059]
                      tunnel: w9943 -> [w10057]
                      tunnel: [w10043] -> w10034
                      tunnel: [w10058] -> w10033
                      tunnel: w9942 -> [_]
                      tunnel: [w10062] -> w10032
                      tunnel: [w10042] -> w10031
                      tunnel: [w10041] -> w10030
                      tunnel: [w10039] -> w10029
                      tunnel: w9941 -> [w10042]
                      tunnel: w9940 -> [w10041]
                      tunnel: ["Where BREAKDOWN_DATE between '%s'and '%s' and BREAKDOWN_STK_HOLD_ID ='%d' and  SHIFT_ID = '%d' and STATION_ID_CID_TRIGGER =%d  "] -> w10028
                      tunnel: [w10039] -> w10027
                      tunnel: w9935 -> [w10037]
                      tunnel: [1 ("BREAKDOWN_STK_HOLD_ID")] -> w9934
                      tunnel: w10034 -> [w10124]
                      tunnel: w10033 -> [w10126]
                      tunnel: w10032 -> [w10121]
                      tunnel: w10031 -> [w10120]
                      tunnel: w10030 -> [w10119]
                      tunnel: [w10123] -> w10026
                      tunnel: [w10125] -> w10025
                      tunnel: [w10121] -> w10024
                      tunnel: [w10111] -> w10023
                      tunnel: [w10117] -> w10022
                      tunnel: [w10120] -> w10021
                      tunnel: [w10119] -> w10020
                      tunnel: w10029 -> [w10116]
                      tunnel: [w10116] -> w10019
                      tunnel: w10028 -> [w10113]
                      tunnel: [w10113] -> w10018
                      tunnel: [w10112] -> w10017
                      tunnel: w10027 -> [w10112]
                      tunnel: w9935 -> [w10110]
                      tunnel: [w10110] -> w9939
                      tunnel: w9934 -> [w10109]
                      tunnel: [w10109] -> w9933
                      tunnel: w10026 -> [w10143]
                      tunnel: w10025 -> [w10141]
                      tunnel: w10024 -> [w10146]
                      tunnel: w10023 -> [w10145]
                      tunnel: w10022 -> [w10144]
                      tunnel: w10021 -> [w10138]
                      tunnel: w10020 -> [w10137]
                      tunnel: [w10146] -> w10016
                      tunnel: [w10145] -> w10015
                      tunnel: [w10144] -> w10014
                      tunnel: [w10142] -> w10013
                      tunnel: [w10135] -> w10012
                      tunnel: [w10134] -> w10011
                      tunnel: [w10139] -> w10010
                      tunnel: [w10138] -> w10009
                      tunnel: [w10137] -> w10008
                      tunnel: w10019 -> [w10133]
                      tunnel: [w10133] -> w10007
                      tunnel: w10018 -> [w10130]
                      tunnel: [w10130] -> w10006
                      tunnel: [w10129] -> w10005
                      tunnel: w10017 -> [w10129]
                      tunnel: w9939 -> [w10128]
                      tunnel: [w10128] -> w9938
                      tunnel: w9933 -> [w10127]
                      tunnel: [w10127] -> w9932
                      tunnel: w10016 -> [w10168]
                      tunnel: w10015 -> [w10167]
                      tunnel: w10014 -> [w10166]
                      tunnel: w10013 -> [w10162]
                      tunnel: w10012 -> [w10165]
                      tunnel: w10011 -> [w10164]
                      tunnel: w10010 -> [w10160]
                      tunnel: w10009 -> [w10158]
                      tunnel: w10008 -> [w10157]
                      tunnel: [w10168] -> w10004
                      tunnel: [w10167] -> w10003
                      tunnel: [w10166] -> w10002
                      tunnel: [w10165] -> w10001
                      tunnel: [w10164] -> w10000
                      tunnel: [w10161] -> w9999
                      tunnel: [w10155] -> w9998
                      tunnel: [w10154] -> w9997
                      tunnel: [w10159] -> w9996
                      tunnel: [w10158] -> w9995
                      tunnel: [w10157] -> w9994
                      tunnel: w10007 -> [w10153]
                      tunnel: [w10153] -> w9993
                      tunnel: w10006 -> [w10150]
                      tunnel: [w10150] -> w9992
                      tunnel: [w10149] -> w9991
                      tunnel: w10005 -> [w10149]
                      tunnel: w9938 -> [w10148]
                      tunnel: [w10148] -> w9937
                      tunnel: w9932 -> [w10147]
                      tunnel: [w10147] -> w9931
                      tunnel: w10004 -> [w10192]
                      tunnel: w10003 -> [w10191]
                      tunnel: w10002 -> [w10190]
                      tunnel: w10001 -> [w10189]
                      tunnel: w10000 -> [w10188]
                      tunnel: w9999 -> [w10184]
                      tunnel: w9998 -> [w10187]
                      tunnel: w9997 -> [w10186]
                      tunnel: w9996 -> [w10183]
                      tunnel: w9995 -> [w10180]
                      tunnel: w9994 -> [w10179]
                      tunnel: [w10192] -> w9990
                      tunnel: [w10191] -> w9989
                      tunnel: [w10190] -> w9988
                      tunnel: [w10189] -> w9987
                      tunnel: [w10188] -> w9986
                      tunnel: [w10187] -> w9985
                      tunnel: [w10186] -> w9984
                      tunnel: [w10182] -> w9983
                      tunnel: [w10181] -> w9982
                      tunnel: [w10177] -> w9981
                      tunnel: [w10176] -> w9980
                      tunnel: [w10180] -> w9979
                      tunnel: [w10179] -> w9978
                      tunnel: w9993 -> [w10175]
                      tunnel: [w10175] -> w9977
                      tunnel: w9992 -> [w10172]
                      tunnel: [w10172] -> w9976
                      tunnel: [w10171] -> w9975
                      tunnel: w9991 -> [w10171]
                      tunnel: w9937 -> [w10170]
                      tunnel: [w10170] -> w9936
                      tunnel: w9931 -> [w10169]
                      tunnel: [w10169] -> w9930
                      tunnel: w9990 -> [w10218]
                      tunnel: w9989 -> [w10217]
                      tunnel: w9988 -> [w10216]
                      tunnel: w9987 -> [w10215]
                      tunnel: w9986 -> [w10214]
                      tunnel: w9985 -> [w10213]
                      tunnel: w9984 -> [w10212]
                      tunnel: w9983 -> [w10206]
                      tunnel: w9982 -> [w10208]
                      tunnel: w9981 -> [w10211]
                      tunnel: w9980 -> [w10210]
                      tunnel: w9979 -> [w10203]
                      tunnel: w9978 -> [w10204]
                      tunnel: [w10218] -> w9974
                      tunnel: [w10217] -> w9973
                      tunnel: [w10216] -> w9972
                      tunnel: [w10215] -> w9971
                      tunnel: [w10214] -> w9970
                      tunnel: [w10213] -> w9969
                      tunnel: [w10212] -> w9968
                      tunnel: [w10211] -> w9967
                      tunnel: [w10210] -> w9966
                      tunnel: [w10207] -> w9965
                      tunnel: [w10205] -> w9964
                      tunnel: [w10201] -> w9963
                      tunnel: [w10199] -> w9962
                      tunnel: w9977 -> [w10200]
                      tunnel: w9976 -> [w10196]
                      tunnel: [w10195] -> w9961
                      tunnel: w9975 -> [w10195]
                      tunnel: w9936 -> [w10194]
                      tunnel: w9930 -> [w10193]
                      tunnel: w9974 -> [w10245]
                      tunnel: w9973 -> [w10238]
                      tunnel: w9972 -> [w10229]
                      tunnel: w9971 -> [w10237]
                      tunnel: w9970 -> [w10227]
                      tunnel: w9969 -> [w10236]
                      tunnel: w9968 -> [w10225]
                      tunnel: w9967 -> [w10235]
                      tunnel: w9966 -> [w10223]
                      tunnel: w9965 -> [w10259]
                      tunnel: w9964 -> [w10258]
                      tunnel: w9963 -> [w10234]
                      tunnel: w9962 -> [w10221]
                      tunnel: [w10259] -> w9960
                      tunnel: [w10258] -> w9959
                      tunnel: [w10252] -> w9958
                      tunnel: [w10245] -> w9957
                      tunnel: [w10244] -> w9956
                      tunnel: [w10243] -> w9955
                      tunnel: [w10242] -> w9954
                      tunnel: [w10241] -> w9953
                      tunnel: [w10240] -> w9952
                      tunnel: [w10239] -> w9951
                      tunnel: [w10238] -> w9950
                      tunnel: [w10237] -> w9949
                      tunnel: [w10236] -> w9948
                      tunnel: [w10235] -> w9947
                      tunnel: [w10234] -> w9946
                      tunnel: [w10219] -> w9945
                      tunnel: w9961 -> [w10219]
                      tunnel: [w10279] -> w9921
                      tunnel: [w10265] -> w9919
                      tunnel: w9960 -> [w10266]
                      tunnel: w9959 -> [w10279]
                      tunnel: w9958 -> [w10264]
                      tunnel: w9957 -> [w10277]
                      tunnel: w9956 -> [w10275]
                      tunnel: w9955 -> [w10273]
                      tunnel: w9954 -> [w10271]
                      tunnel: w9953 -> [w10269]
                      tunnel: w9952 -> [w10267]
                      tunnel: w9951 -> [w10260]
                      tunnel: w9950 -> [w10276]
                      tunnel: w9949 -> [w10274]
                      tunnel: w9948 -> [w10272]
                      tunnel: w9947 -> [w10270]
                      tunnel: w9946 -> [w10268]
                      tunnel: w9945 -> [w10263]
                      tunnel: [w10260] -> w9929
                      frame #0 {
                        w10050 = "%Y-%m-%d" ("time format string (%c)")
                        n1816 = Decimal String To Number(string=w10037) -> (number=w10036:i32)  [unwired: 2 in, 1 out]
                        n1817 = property on="Table" class="Tbl (strict)"("Visible"=TRUE) -> ()  [unwired: 2 in, 2 out]
                        n1818 = Format Date/Time String(time format string (%c)=w10050, seconds (now)=w10042) -> (date/time string=w10051:string)  [unwired: 1 in]
                        n1819 = Format Date/Time String(time format string (%c)=w10050, seconds (now)=w10041) -> (date/time string=w10049:string)  [unwired: 1 in]
                        n1820 = Format Into String(format string="Where BREAKDOWN_DATE between '%s' and '%s' and  SHIFT_ID = '%d'  ", w10051, w10049, w10036) -> (resulting string=w10048:string)  [unwired: 2 in, 1 out]
                        n1821 = call <vilib>:"DB Tools Select Data.vi"("condition"=w10048, "error in (no error)"=w10057, "columns"=string[] ["BREAKDOWN_DATE"], "table"="STATION_1_LOG_HISTORY", "connection reference"=w10059) -> ("error out"=w10044:errorcluster, "data"=w10047:variant[][], "connection reference out"=w10058:T2)  [unwired: 1 in]
                        n1822 = property on="Table 2" class="Tbl (strict)"("Visible"=FALSE) -> ()  [unwired: 2 in, 2 out]
                        n1823 = xnode "Database Variant To Data"("database variant"=w10047, "error in (no error)"=w10044, "type"=string[][] [] ("Elements Found")) -> ("data"=w10045:string[][], "error out"=w10043:errorcluster)
                        n1824 = Index Array(array=w10045, index (col)=0 ("disabled index (col)")) -> (element=w10053:string[])  [unwired: 1 in]
                        n1825 = call "Search_1d_array_element.vi"("Count in"=string[] [] ("Elements Found"), "BD Date"=w10053, "Elements Found in"=string[] [] ("Elements Found")) -> ("Elements Found out"=w10039:string[])  [unwired: 4 in, 2 out]
                        n1826 = Build Array(w10039) -> (w10063:string[][])
                        n1827 = Transpose 2D Array(2D array=w10063) -> (transposed array=w10062:string[][])
                      }
                      frame #1 {
                        n1828 = call "Stack_holderwise_total_bd_count_&_duration_3_for_stationwise.vi"("Refnum in"=w10126, "BREAKDOWN_STK_HOLD_ID"=1, "condition"=w10113, "Form Date"=w10120, "To Date"=w10119, "error in (no error)"=w10124, "STATION_ID_CID_TRIGGER"=w10109, "Shift"=w10110) -> ("Refnum out"=w10125:T2, "Count out"=w10118:string[], "appended array"=w10115:dbl[], "error out"=w10123:errorcluster)  [unwired: 4 in]
                        n1829 = call "NUMERIC TO STRING.vi"("appended array"=w10115) -> ("Array"=w10114:string[])  [unwired: 4 in]
                        n1830 = call "Insert_empty_element_with_zero.vi"("searched date"=w10118, "fixed date"=w10116) -> ("O/P"=w10111:string[])  [unwired: 9 in]
                        n1831 = call "Insert_empty_element_with_zero.vi"("searched date"=w10114, "fixed date"=w10116) -> ("O/P"=w10117:string[])  [unwired: 9 in]
                      }
                      frame #2 {
                        n1832 = call "Stack_holderwise_total_bd_count_&_duration_3_for_stationwise.vi"("Refnum in"=w10141, "BREAKDOWN_STK_HOLD_ID"=2, "condition"=w10130, "Form Date"=w10138, "To Date"=w10137, "error in (no error)"=w10143, "STATION_ID_CID_TRIGGER"=w10127, "Shift"=w10128) -> ("Refnum out"=w10139:T2, "Count out"=w10136:string[], "appended array"=w10132:dbl[], "error out"=w10142:errorcluster)  [unwired: 4 in]
                        n1833 = call "Insert_empty_element_with_zero.vi"("searched date"=w10136, "fixed date"=w10133) -> ("O/P"=w10135:string[])  [unwired: 9 in]
                        n1834 = call "NUMERIC TO STRING.vi"("appended array"=w10132) -> ("Array"=w10131:string[])  [unwired: 4 in]
                        n1835 = call "Insert_empty_element_with_zero.vi"("searched date"=w10131, "fixed date"=w10133) -> ("O/P"=w10134:string[])  [unwired: 9 in]
                      }
                      frame #3 {
                        n1836 = call "Stack_holderwise_total_bd_count_&_duration_3_for_stationwise.vi"("Refnum in"=w10160, "BREAKDOWN_STK_HOLD_ID"=3, "condition"=w10150, "Form Date"=w10158, "To Date"=w10157, "error in (no error)"=w10162, "STATION_ID_CID_TRIGGER"=w10147, "Shift"=w10148) -> ("Refnum out"=w10159:T2, "Count out"=w10156:string[], "appended array"=w10152:dbl[], "error out"=w10161:errorcluster)  [unwired: 4 in]
                        n1837 = call "Insert_empty_element_with_zero.vi"("searched date"=w10156, "fixed date"=w10153) -> ("O/P"=w10155:string[])  [unwired: 9 in]
                        n1838 = call "NUMERIC TO STRING.vi"("appended array"=w10152) -> ("Array"=w10151:string[])  [unwired: 4 in]
                        n1839 = call "Insert_empty_element_with_zero.vi"("searched date"=w10151, "fixed date"=w10153) -> ("O/P"=w10154:string[])  [unwired: 9 in]
                      }
                      frame #4 {
                        n1840 = call "Stack_holderwise_total_bd_count_&_duration_3_for_stationwise.vi"("Refnum in"=w10183, "BREAKDOWN_STK_HOLD_ID"=4, "condition"=w10172, "Form Date"=w10180, "To Date"=w10179, "error in (no error)"=w10184, "STATION_ID_CID_TRIGGER"=w10169, "Shift"=w10170) -> ("Refnum out"=w10182:T2, "Count out"=w10178:string[], "appended array"=w10174:dbl[], "error out"=w10181:errorcluster)  [unwired: 4 in]
                        n1841 = call "Insert_empty_element_with_zero.vi"("searched date"=w10178, "fixed date"=w10175) -> ("O/P"=w10177:string[])  [unwired: 9 in]
                        n1842 = call "NUMERIC TO STRING.vi"("appended array"=w10174) -> ("Array"=w10173:string[])  [unwired: 4 in]
                        n1843 = call "Insert_empty_element_with_zero.vi"("searched date"=w10173, "fixed date"=w10175) -> ("O/P"=w10176:string[])  [unwired: 9 in]
                      }
                      frame #5 {
                        n1844 = call "Stack_holderwise_total_bd_count_&_duration_3_for_stationwise.vi"("Refnum in"=w10206, "BREAKDOWN_STK_HOLD_ID"=5, "condition"=w10196, "Form Date"=w10203, "To Date"=w10204, "error in (no error)"=w10208, "STATION_ID_CID_TRIGGER"=w10193, "Shift"=w10194) -> ("Refnum out"=w10205:T2, "Count out"=w10202:string[], "appended array"=w10198:dbl[], "error out"=w10207:errorcluster)  [unwired: 4 in]
                        n1845 = call "NUMERIC TO STRING.vi"("appended array"=w10198) -> ("Array"=w10197:string[])  [unwired: 4 in]
                        n1846 = call "Insert_empty_element_with_zero.vi"("searched date"=w10202, "fixed date"=w10200) -> ("O/P"=w10201:string[])  [unwired: 9 in]
                        n1847 = call "Insert_empty_element_with_zero.vi"("searched date"=w10197, "fixed date"=w10200) -> ("O/P"=w10199:string[])  [unwired: 9 in]
                      }
                      frame #6 {
                        n1848 = call "String to numeric.vi"("Array"=w10229) -> ("Array 2"=w10228:dbl[])  [unwired: 4 in]
                        n1849 = call "String to numeric.vi"("Array"=w10227) -> ("Array 2"=w10226:dbl[])  [unwired: 4 in]
                        n1850 = call "String to numeric.vi"("Array"=w10225) -> ("Array 2"=w10224:dbl[])  [unwired: 4 in]
                        n1851 = call "String to numeric.vi"("Array"=w10223) -> ("Array 2"=w10222:dbl[])  [unwired: 4 in]
                        n1852 = call "String to numeric.vi"("Array"=w10221) -> ("Array 2"=w10220:dbl[])  [unwired: 4 in]
                        n1853 = Decimal String To Number(string=w10234) -> (number=w10253:i32[])  [unwired: 2 in, 1 out]
                        n1854 = Decimal String To Number(string=w10235) -> (number=w10254:i32[])  [unwired: 2 in, 1 out]
                        n1855 = Decimal String To Number(string=w10236) -> (number=w10255:i32[])  [unwired: 2 in, 1 out]
                        n1856 = Decimal String To Number(string=w10237) -> (number=w10256:i32[])  [unwired: 2 in, 1 out]
                        n1857 = Decimal String To Number(string=w10238) -> (number=w10251:i32[])  [unwired: 2 in, 1 out]
                        n1858 = Compound Arithmetic op=ADD(w10228, w10226, w10224, w10222, w10220) -> (w10231:dbl[])
                        n1859 = Build Array(w10229) -> (w10250:string[][])
                        n1860 = Build Array(w10227) -> (w10249:string[][])
                        n1861 = Build Array(w10225) -> (w10248:string[][])
                        n1862 = Build Array(w10223) -> (w10247:string[][])
                        n1863 = Build Array(w10221) -> (w10246:string[][])
                        n1864 = Number To Fractional String(number=w10231, precision (6)=i16 2) -> (F-format string=w10230:string[])  [unwired: 2 in]
                        n1865 = Compound Arithmetic op=ADD(w10253, w10254, w10255, w10256, w10251) -> (w10257:i32[])
                        n1866 = Transpose 2D Array(2D array=w10250) -> (transposed array=w10244:string[][])
                        n1867 = Transpose 2D Array(2D array=w10249) -> (transposed array=w10243:string[][])
                        n1868 = Transpose 2D Array(2D array=w10248) -> (transposed array=w10242:string[][])
                        n1869 = Transpose 2D Array(2D array=w10247) -> (transposed array=w10241:string[][])
                        n1870 = Transpose 2D Array(2D array=w10246) -> (transposed array=w10240:string[][])
                        n1871 = Number To Decimal String(number=w10257) -> (decimal integer string=w10252:string[])  [unwired: 1 in]
                        n1872 = Build Array(w10230) -> (w10233:string[][])
                        n1873 = Transpose 2D Array(2D array=w10233) -> (transposed array=w10239:string[][])
                      }
                      frame #7 {
                        n1874 = Insert Into Array(array=w10277, index (col)=1 ("disabled index (col)"), new element #1=w10276, new element #2=w10275, new element #3=w10274, new element #4=w10273, new element #5=w10272, new element #6=w10271, new element #7=w10270, new element #8=w10269, new element #9=w10268, new element #10=w10267, new element #11=w10264, new element #12=w10260) -> (w10262:string[][])  [unwired: 1 in]
                        n1875 = call "flot graph for month n year.vi"("BD Date"=w10263, "error in (no error)"=w10266, "Count total"=w10264) -> ("error out"=w10265:errorcluster, "Run-Time Status"=w10261:cluster{"Array 2":timestamp[], dbl[]})  [unwired: 7 in]
                        n1876 = local write "Run-Time Status"(w10261) -> ()
                        n1877 = local write "Table"(w10262) -> ()
                      }
                    }
                    n1878 = call "OEE_PART_1.vi"("CYCLE TIME"=w9927, "ACTUAL PROD TIME"=w9928, "BREAKDOWN TOTAL TIME"=w9929) -> ("Numeric"=w9914:i32, "CAPACITY"=w9913:dbl, "ACTUAL TIME"=w9915:i32)  [unwired: 5 in, 1 out]
                    n1879 = call "OEE_PART_2_P.vi"("Refnum in"=w9921, "Shift"=w9925, "String"="ALL", "Select Station"=w9922, "Form Date"=w9924, "To Date"=w9923, "AVAILABLILITY TIME"=w9915, "CAPACITY"=w9913) -> ("Refnum out"=w9920:T2, "QUALITY"=w9918:dbl, "OEE"=w9916:dbl, "PERFORMANCE"=w9917:dbl)  [unwired: 2 in, 2 out]
                    n1880 = local write "PERFORMANCE"(w9917) -> ()
                    n1881 = local write "QUALITY"(w9918) -> ()
                    n1882 = local write "OEE"(w9916) -> ()
                    n1883 = local write "AVAILABLILITY TIME(MIN)"(w9915) -> ()
                    n1884 = local write "IDEAL CYCLE TIME"(w9914) -> ()
                    n1885 = local write "CAPACITY"(w9913) -> ()
                  }
                  frame "3" {
                    n1886 = flat-sequence {
                      tunnel: w10311 -> [w10426]
                      tunnel: w10310 -> [w10424]
                      tunnel: [w10410] -> w10401
                      tunnel: [w10425] -> w10400
                      tunnel: w10309 -> [_]
                      tunnel: [w10429] -> w10399
                      tunnel: [w10409] -> w10398
                      tunnel: [w10408] -> w10397
                      tunnel: [w10406] -> w10396
                      tunnel: w10308 -> [w10409]
                      tunnel: w10307 -> [w10408]
                      tunnel: ["Where BREAKDOWN_DATE between '%s'and '%s' and BREAKDOWN_STK_HOLD_ID ='%d' and  SHIFT_ID = '%d' and STATION_ID_CID_TRIGGER =%d  "] -> w10395
                      tunnel: [w10406] -> w10394
                      tunnel: w10302 -> [w10404]
                      tunnel: [1 ("BREAKDOWN_STK_HOLD_ID")] -> w10301
                      tunnel: w10401 -> [w10491]
                      tunnel: w10400 -> [w10493]
                      tunnel: w10399 -> [w10488]
                      tunnel: w10398 -> [w10487]
                      tunnel: w10397 -> [w10486]
                      tunnel: [w10490] -> w10393
                      tunnel: [w10492] -> w10392
                      tunnel: [w10488] -> w10391
                      tunnel: [w10478] -> w10390
                      tunnel: [w10484] -> w10389
                      tunnel: [w10487] -> w10388
                      tunnel: [w10486] -> w10387
                      tunnel: w10396 -> [w10483]
                      tunnel: [w10483] -> w10386
                      tunnel: w10395 -> [w10480]
                      tunnel: [w10480] -> w10385
                      tunnel: [w10479] -> w10384
                      tunnel: w10394 -> [w10479]
                      tunnel: w10302 -> [w10477]
                      tunnel: [w10477] -> w10306
                      tunnel: w10301 -> [w10476]
                      tunnel: [w10476] -> w10300
                      tunnel: w10393 -> [w10510]
                      tunnel: w10392 -> [w10508]
                      tunnel: w10391 -> [w10513]
                      tunnel: w10390 -> [w10512]
                      tunnel: w10389 -> [w10511]
                      tunnel: w10388 -> [w10505]
                      tunnel: w10387 -> [w10504]
                      tunnel: [w10513] -> w10383
                      tunnel: [w10512] -> w10382
                      tunnel: [w10511] -> w10381
                      tunnel: [w10509] -> w10380
                      tunnel: [w10502] -> w10379
                      tunnel: [w10501] -> w10378
                      tunnel: [w10506] -> w10377
                      tunnel: [w10505] -> w10376
                      tunnel: [w10504] -> w10375
                      tunnel: w10386 -> [w10500]
                      tunnel: [w10500] -> w10374
                      tunnel: w10385 -> [w10497]
                      tunnel: [w10497] -> w10373
                      tunnel: [w10496] -> w10372
                      tunnel: w10384 -> [w10496]
                      tunnel: w10306 -> [w10495]
                      tunnel: [w10495] -> w10305
                      tunnel: w10300 -> [w10494]
                      tunnel: [w10494] -> w10299
                      tunnel: w10383 -> [w10535]
                      tunnel: w10382 -> [w10534]
                      tunnel: w10381 -> [w10533]
                      tunnel: w10380 -> [w10529]
                      tunnel: w10379 -> [w10532]
                      tunnel: w10378 -> [w10531]
                      tunnel: w10377 -> [w10527]
                      tunnel: w10376 -> [w10525]
                      tunnel: w10375 -> [w10524]
                      tunnel: [w10535] -> w10371
